vi "251201_Nikon_CheckStatus_PFS.vi"(8 "error in":errorcluster caption="entrée d'erreur", 11 "NikonTi2AxLib.INikonTi2AxMicroscope":refnum<k7>) -> (0 "error out":errorcluster={"status"=TRUE, "code"=-9, "source"="Exception occured in Nikon.Ti2.Microscope.1: Failed in 231026_NikonTi2_Indicators_v2.vi"} caption="sortie d'erreur", 2 "PFS cluster":T1, 3 "reference out":refnum<k7>)   [LabVIEW 2025]
doc: "This vi checks the current status of the microscope. One can add some extra devices such as fluorescence cube turret.\nThe automation should be open and close outside of this vi"
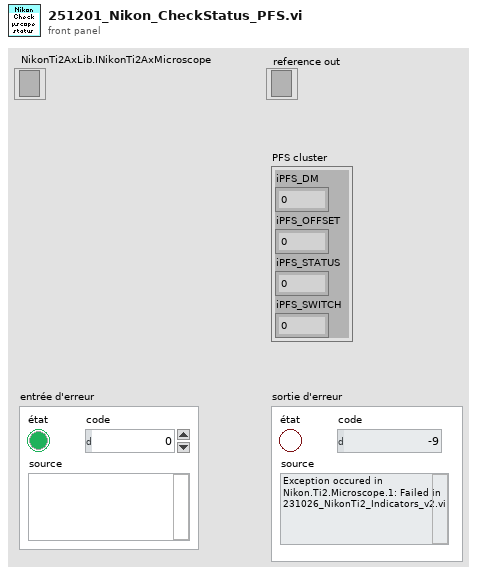
[diagram p1: front panel]
types:
  T1 = cluster{"iPFS_DM":i32, "iPFS_OFFSET":i32, "iPFS_STATUS":i32, "iPFS_SWITCH":i32}
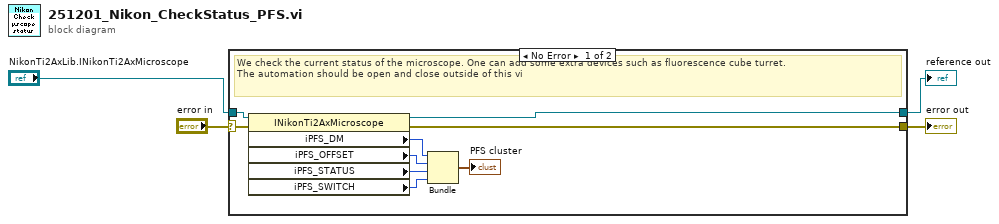
[diagram p0: block diagram]
diagram:
  n1 = case shown="No Error" "error in" {
    selector: "error in" -> [w12 w15]
    tunnel: [w11 w15] -> w3
    tunnel: "NikonTi2AxLib.INikonTi2AxMicroscope" -> [w13 w14]
    tunnel: [w10 w14] -> w2
    frame No Error {
      # "We check the current status of the microscope. One can add some extra devices such as fluorescence cube turret.\nThe automation should be open and close outside of this vi"
      n2 = property class="INikonTi2AxMicroscope"(reference=w13, error in=w12) -> (reference out=w10:refnum<k7>, error out=w11:errorcluster, "iPFS_DM"=w9:i32, "iPFS_OFFSET"=w8:i32, "iPFS_STATUS"=w7:i32, "iPFS_SWITCH"=w6:i32)
      n3 = Bundle("iPFS_DM"=w9, "iPFS_OFFSET"=w8, "iPFS_STATUS"=w7, "iPFS_SWITCH"=w6) -> (→"PFS cluster":T1)  [unwired: 1 in]
    }
    frame Error {
    }
  }
  "error out" <- w3
  "reference out" <- w2
